vi "Close.vi"(8 "error in (no error)":errorcluster {"code" format="%x"}) -> (0 "error out":errorcluster {"code" format="%x"})   [LabVIEW 8.6, in "Keyence LK-G5000.lvlib"]
doc: "Performs an instrument error query before terminating the software connection to the instrument."
uses:
  Keyence LK-G5000.lvlib
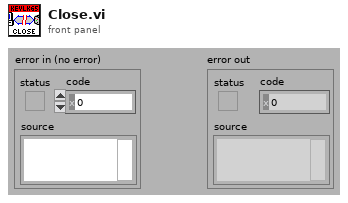
[diagram p1: front panel]
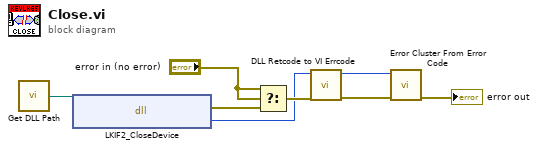
[diagram p0: block diagram]
diagram:
  n1 = call "Get DLL Path.vi"() -> ("DLL Path"=w1:path)  [unwired: 1 in]
  n2 = dll-call lib="C:/Program Files/National Instruments/LabVIEW 2011/instr.lib/Keyence LK-G5000/LKIF2.dll" fn="LKIF2_CloseDevice"(path in=w1) -> (error out=w8:errorcluster, "RC"=w5:i32)  [unwired: 2 in, 1 out]
  n3 = Select(t="error in (no error)", s="error in (no error)", f=w8) -> (s? t:f=w6:errorcluster)
  n4 = call "DLL Retcode to VI Errcode.vi"("error in (no error)"=w6, "DLL Retcode"=w5) -> ("error out"=w3:errorcluster, "VI Errcode"=w4:i32)  [unwired: 8 in]
  n5 = call <vilib>:"Error Cluster From Error Code.vi"("error in (no error)"=w3, "error code (0)"=w4) -> ("error out"=→"error out":errorcluster)  [unwired: 7 in]
